vi "Calculate Acceptance Probability.vi"(8 "error in (no error)":errorcluster, 11 "SA in":refnum<class "SA.lvclass">) -> (0 "error out":errorcluster, 2 "Acceptance Probability":dbl, 3 "SA out":refnum<class "SA.lvclass">)   [LabVIEW 2013, in "SA.lvclass"]
uses:
  SA.lvclass
  SA.lvclass/SA.ctl
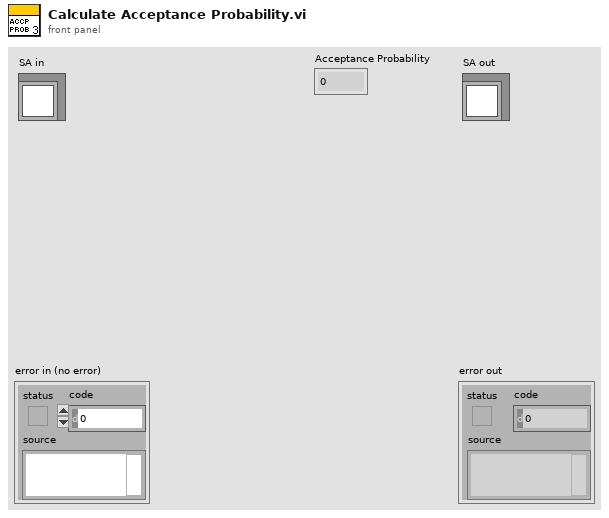
[diagram p1: front panel]
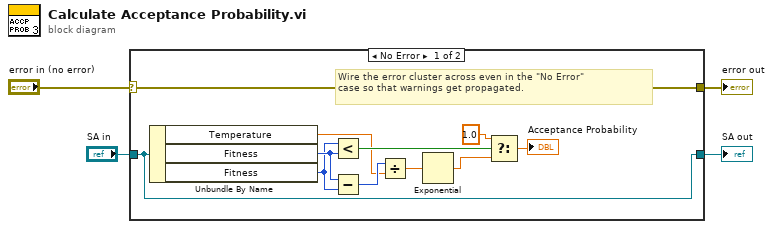
[diagram p0: block diagram]
diagram:
  n1 = case shown="No Error" "error in (no error)" {
    selector: "error in (no error)" -> [w15 w17]
    tunnel: [w15 w17] -> w3
    tunnel: [w14 w16] -> w1
    tunnel: "SA in" -> [w14 w16]
    frame No Error {
      # "Wire the error cluster across even in the \"No Error\"\ncase so that warnings get propagated."
      n2 = Unbundle By Name(w14) -> ("Temperature"=w8:dbl, "Fitness"=w11:u16, "Fitness"=w10:u16)
      n3 = Less?(x=w10, y=w11) -> (x < y?=w13:bool)
      n4 = Subtract(x=w11, y=w10) -> (x-y=w9:u16)
      n5 = Divide(x=w9, y=w8) -> (x/y=w7:dbl)
      n6 = Exponential(1:w7) -> (0:w6:dbl)
      n7 = Select(t=1.0, s=w13, f=w6) -> (s? t:f=→"Acceptance Probability":dbl)
    }
    frame Error {
    }
  }
  "error out" <- w3
  "SA out" <- w1
